vi "decodeStream.vi"(8 "error in (no error)":errorcluster, 9 "beginIndex":i32, 10 "binary stream":u8[](array[numeric]), 11 "tBSONNull in":refnum<class "tBSONNull.lvclass">) -> (0 "error out":errorcluster, 1 "endIndex":i32, 2 "binary stream out":u8[](array[numeric]), 3 "tBSONNull out":refnum<class "tBSONNull.lvclass">)   [LabVIEW 2013, in "BSON.lvlib" / "tBSONNull.lvclass"]
uses:
  tBSONNull.lvclass
  tBSONElement/tBSONElement.lvclass
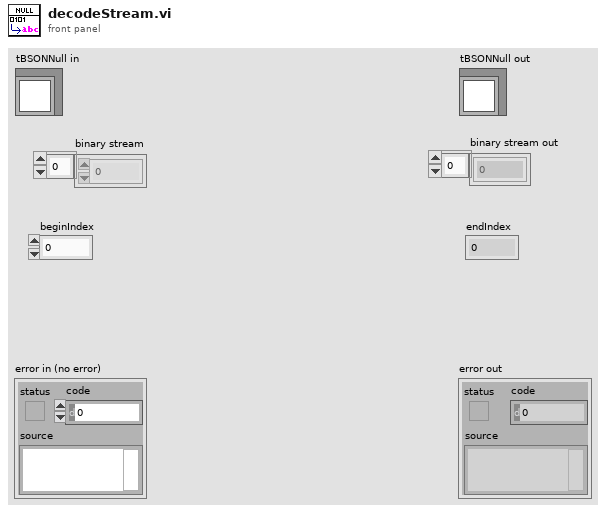
[diagram p1: front panel]
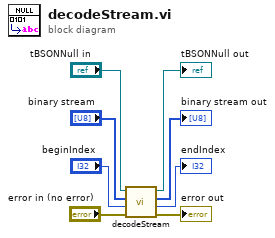
[diagram p0: block diagram]
diagram:
  n1 = call-parent "decodeStream.vi"("error in (no error)"="error in (no error)", "beginIndex"="beginIndex", "binary stream"="binary stream", "tBSONElement in"="tBSONNull in") -> ("error out"=→"error out":errorcluster, "endIndex"=→"endIndex":i32, "binary stream out"=→"binary stream out":u8[], "tBSONElement out"=→"tBSONNull out":refnum<class "tBSONNull.lvclass">)  [unwired: 4 in]
